vi "4_6 Light Intensity Meter using Photocell.vi"() -> ()   [LabVIEW 2025]
uses:
  <vilib>/express/express arith-compare/Formula/XNode/ExpressFormulaBlockNode.xnode
panel:
  in  "stop":bool
  out "Alarm":bool
  out "Warning":bool
  out "Light Intensity Graph":dbl(graph)
  in  "Light Intensity Threshold in kohms":dbl(knob) scale=0.0..100.0
  out "Voltage Reading":dbl(knob) scale=0.0..5.0
  out "Photocell resistance Kohoms":dbl(knob) scale=0.0..100.0
  in  "Photocell voltage":dbl(knob) scale=0.0..5.0
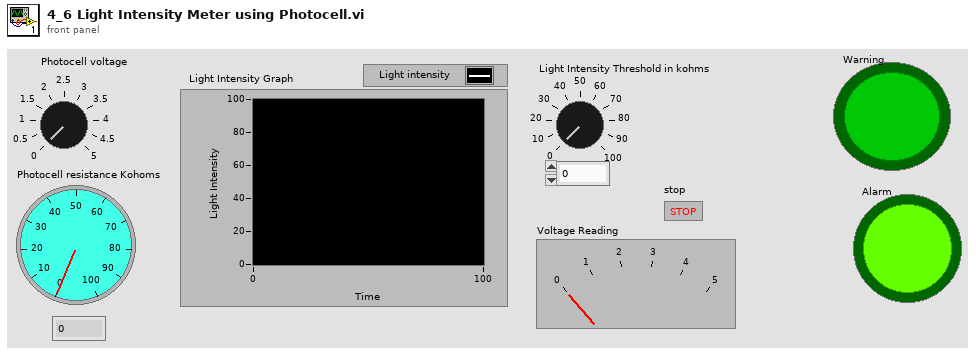
[diagram p1: front panel]
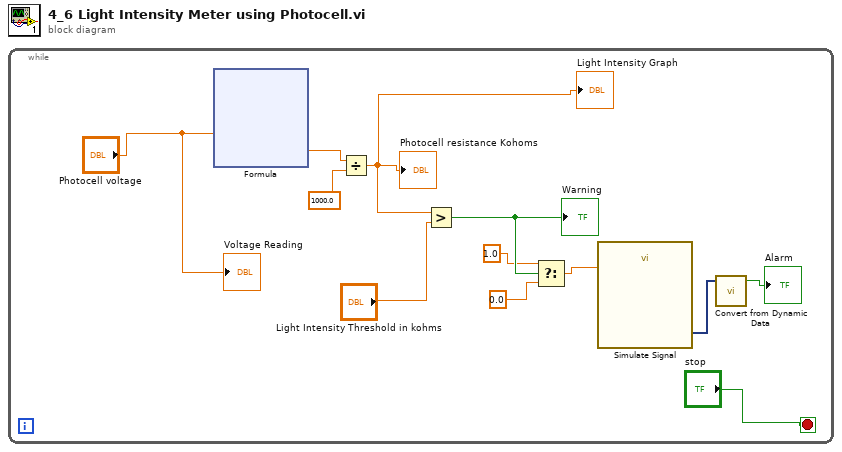
[diagram p0: block diagram]
diagram:
  n1 = while {
    stop <- "stop" stop-if-true
    n2 = xnode "Formula"("V"="Photocell voltage") -> ("Result"=w11:dbl)  [unwired: 1 in, 1 out]
    n3 = Divide(x=w11, y=1000.0) -> (x/y=w9:dbl)
    "Photocell resistance Kohoms" <- w9
    "Light Intensity Graph" <- w9
    n4 = Greater?(x=w9, y="Light Intensity Threshold in kohms") -> (0:w5:bool)
    "Warning" <- w5
    n5 = Select(t=1.0, s=w5, f=0.0) -> (s? t:f=w6:dbl)
    n6 = call "Simulate Signal"("Amplitude"=w6) -> ("Square"=w2:dynamicdata)  [unwired: 13 in, 1 out]
    n7 = call "Convert from Dynamic Data"("Dynamic Data Type"=w2) -> ("Scalar"=→"Alarm":bool)  [unwired: 3 in]
    "Voltage Reading" <- "Photocell voltage"
  }
